vi "Data To Variant_I8.vi"(8 "error in (no error)":errorcluster, 11 "Data":i64[](array[numeric])) -> (0 "error out":errorcluster, 3 "Variant":variant)   [LabVIEW 2020, in "SECS Communication.lvlib" / "SECS-II Class.lvclass"]
uses:
  SECS-II Class.lvclass
  SECS-II Class.lvclass/SECS-II Class.ctl
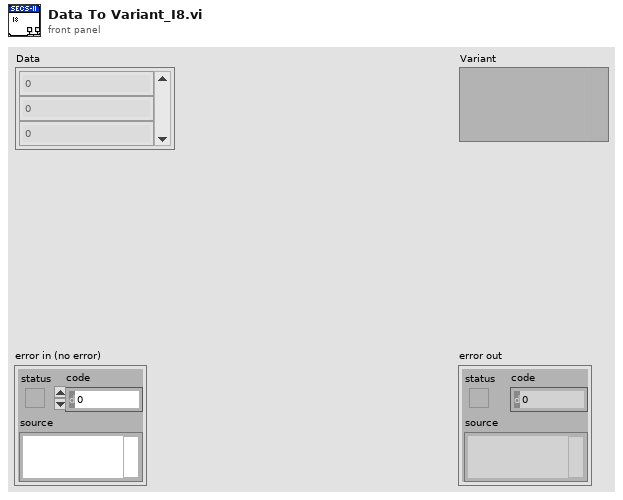
[diagram p1: front panel]
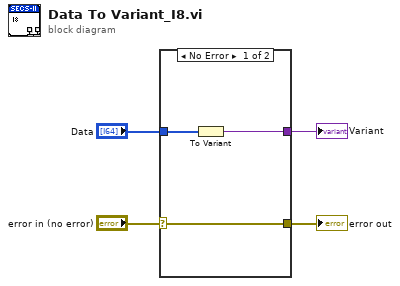
[diagram p0: block diagram]
diagram:
  n1 = case shown="No Error" "error in (no error)" {
    selector: "error in (no error)" -> [w7 w8]
    tunnel: [w7 w8] -> w3
    tunnel: "Data" -> [w6 _]
    tunnel: [w5 _] -> w1
    frame No Error {
      n2 = To Variant(anything=w6) -> (Variant=w5:variant)
    }
    frame Error {
    }
  }
  "error out" <- w3
  "Variant" <- w1
